vi "Check for Empty Command Or Response.vi"(7 "Command/Response Refnum in":T1 format="%.0x", 8 "Error In":errorcluster, 11 "Response Format in":string) -> (0 "Error Out":errorcluster, 3 "Response Format out":string)   [LabVIEW 2020, in "Instrument Addon Scripting API.lvlib"]
uses:
  Instrument Addon Scripting API.lvlib
  <vilib>/NI VeriStand/Custom Device API/Custom Device Item Ref.ctl
  <vilib>/NI VeriStand/Custom Device API/Custom Device API.lvlib
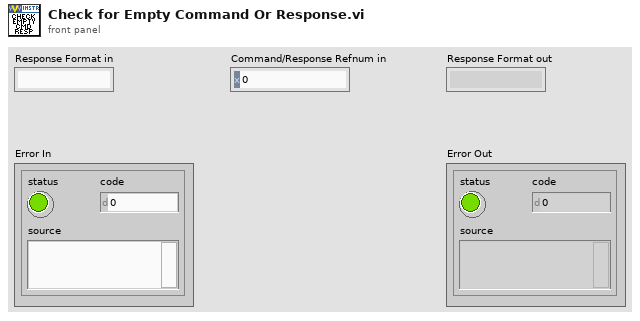
[diagram p1: front panel]
types:
  T1 = typedef "Custom Device API.lvlib/Custom Device Item Ref.ctl" = u64
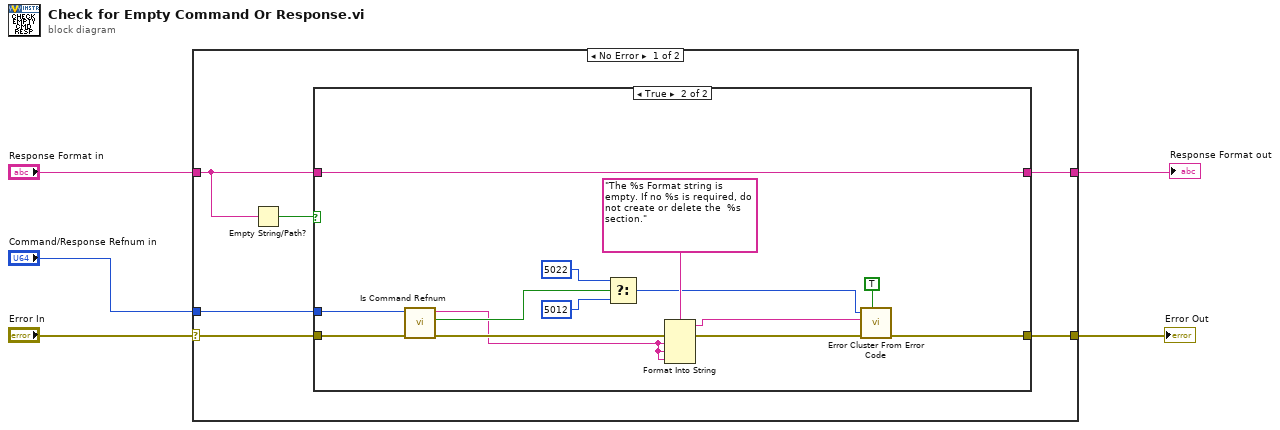
[diagram p0: block diagram]
diagram:
  n1 = case shown="No Error" "Error In" {
    selector: "Error In" -> [w8 w28]
    tunnel: "Response Format in" -> [w10 w29]
    tunnel: [w9 w29] -> w4
    tunnel: [w7 w28] -> w2
    tunnel: "Command/Response Refnum in" -> [w6 _]
    frame No Error {
      n2 = Empty String/Path?(string/path=w10) -> (empty?=w11:bool)
      n3 = case shown="True" w11 {
        tunnel: w10 -> [w13 w27]
        tunnel: [w13 w27] -> w9
        tunnel: w8 -> [w12 w20]
        tunnel: [w12 w26] -> w7
        tunnel: w6 -> [_ w18]
        frame False {
        }
        frame True {
          n4 = call "Is Command Refnum.vi"("error in (no error)"=w20, "Command/Response Refnum in"=w18) -> ("error out"=w24:errorcluster, "Is Command?"=w25:bool, "Command/Response out"=w15:string)  [unwired: 7 in]
          n5 = Select(t=5022 ("error code (0)"), s=w25, f=5012 ("error code (0)")) -> (s? t:f=w17:i32)
          n6 = Format Into String(format string="The %s Format string is empty. If no %s is required, do not create or delete the  %s section." ("error message (\"\")"), error in=w24, w15, w15, w15) -> (resulting string=w16:string, error out=w19:errorcluster)  [unwired: 1 in]
          n7 = call <vilib>:"Error Cluster From Error Code.vi"("show call chain? (False)"=TRUE, "error in (no error)"=w19, "error message (\"\")"=w16, "error code (0)"=w17) -> ("error out"=w26:errorcluster)  [unwired: 5 in]
        }
      }
    }
    frame Error {
    }
  }
  "Response Format out" <- w4
  "Error Out" <- w2
